vi "merFISH_initialize_Z_ramp.vi"(3 "error in":errorcluster, 4 "Total range (nm)":u32, 5 "dZ (nm)":u32) -> (0 "error out":errorcluster, 1 "Total # steps":i32, 2 "Ramp":dbl[](array[numeric]))   [LabVIEW 2015]
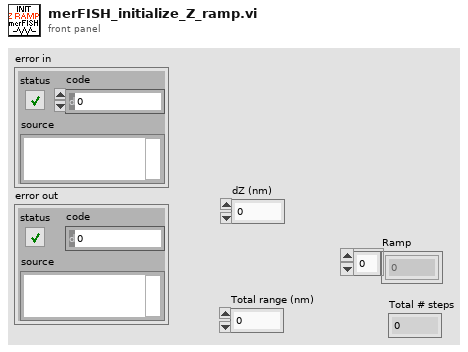
[diagram p1: front panel]
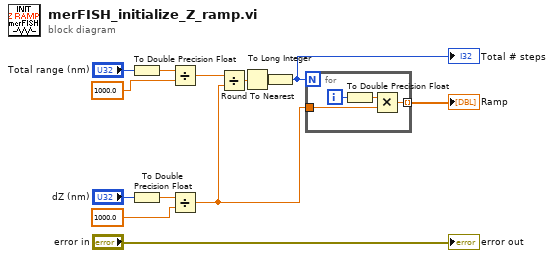
[diagram p0: block diagram]
diagram:
  n1 = To Double Precision Float(number="Total range (nm)") -> (double precision float=w10:dbl)
  n2 = To Double Precision Float(number="dZ (nm)") -> (double precision float=w9:dbl)
  n3 = Divide(x=w10, y=1000.0) -> (x/y=w8:dbl)
  n4 = Divide(x=w9, y=1000.0) -> (x/y=w4:dbl)
  n5 = Divide(x=w8, y=w4) -> (x/y=w2:dbl)
  n6 = Round To Nearest(number=w2) -> (nearest integer value=w1:dbl)
  n7 = To Long Integer(number=w1) -> (32bit integer=w6:i32)
  "Total # steps" <- w6
  n8 = for {
    N: w6 -> [_]
    tunnel: w4 -> [w16]
    tunnel: [w15] -> w5 mode=indexing
    i -> [w17]
    n9 = To Double Precision Float(number=w17) -> (double precision float=w14:dbl)
    n10 = Multiply(x=w14, y=w16) -> (x*y=w15:dbl)
  }
  "Ramp" <- w5
  "error out" <- "error in"
